vi "Rayleigh Random.vi"(6 "seed":i32=-1, 7 "reset":bool, 10 "b":dbl=3.0, 11 "samples":i32=128) -> (0 "error":i32, 3 "Rayleigh random data":dbl[](array[numeric]))   [LabVIEW 2010, in "NI_Gmath.lvlib"]
doc: "Generates random values from a variate X, where X describes the selected distribution type. You must manually select the polymorphic instance to use."
uses:
  NI_Gmath.lvlib
panel:
  # "Rayleigh Random"
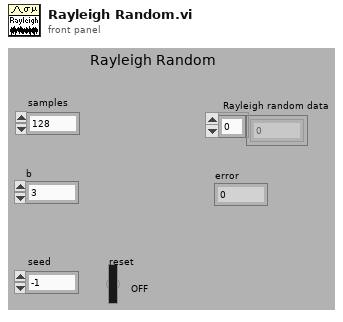
[diagram p1: front panel]
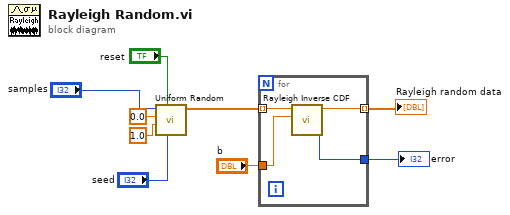
[diagram p0: block diagram]
diagram:
  n1 = call "Uniform Random.vi"("seed"="seed", "reset"="reset", "xmax"=1.0, "xmin"=0.0, "samples"="samples") -> ("uniform random data"=w3:dbl[])  [unwired: 5 in, 1 out]
  n2 = for {
    tunnel: "b" -> [w11]
    tunnel: [w13] -> w8 mode=indexing
    tunnel: [w12] -> w7
    tunnel: w3 -> [w10] mode=indexing
    n3 = call "Rayleigh Inverse CDF.vi"("b"=w11, "cdf(x)"=w10) -> ("error"=w12:i32, "x"=w13:dbl)  [unwired: 8 in]
  }
  "error" <- w7
  "Rayleigh random data" <- w8
